vi "Fgen Module.vi"() -> ()   [LabVIEW 2021]
panel:
  in  "duration":dbl
  out "Actual Duration":dbl
  in  "I2C Generator Fgen":refnum<k15>
  in  "amplitude":dbl=6.0
  in  "frequency":dbl=6.0
  in  "waveform":T1(ring)=enum."Noise"
  in  "I2C Generator Fgen Channel":string
  out "error out":errorcluster
  in  "error in":errorcluster
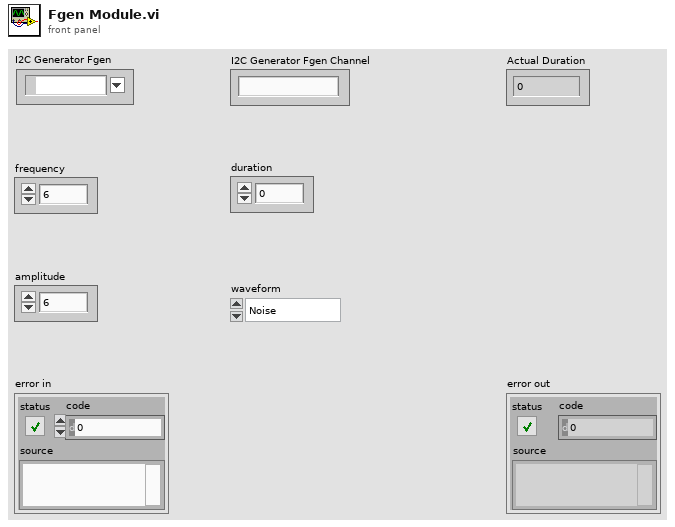
[diagram p1: front panel]
types:
  T1 = enum32{"Sine", "Square", "Triangle", "Ramp Up", "Ramp Down", "DC", "Noise", "User"}
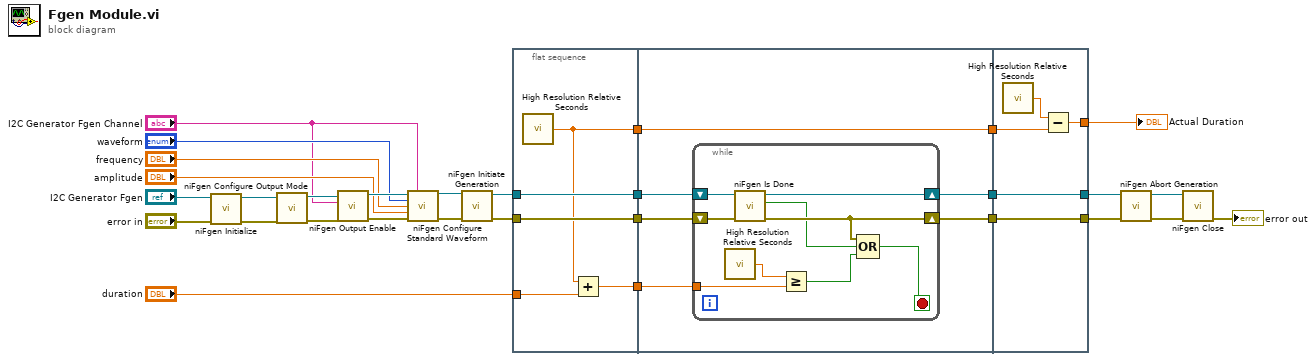
[diagram p0: block diagram]
diagram:
  n1 = call <instrlib>:"niFgen Initialize.vi"("error in (no error)"="error in", "Resource Name"="I2C Generator Fgen") -> ("error out"=w27:errorcluster, "Instrument Handle Out"=w30:refnum<k15>)  [unwired: 8 in]
  n2 = call <instrlib>:"niFgen Configure Output Mode.vi"("error in (no error)"=w27, "Instrument Handle"=w30) -> ("error out"=w15:errorcluster, "Instrument Handle Out"=w26:refnum<k15>)  [unwired: 7 in]
  n3 = call <instrlib>:"niFgen Output Enable.vi"("error in (no error)"=w15, "Channel Name"="I2C Generator Fgen Channel", "Instrument Handle"=w26) -> ("error out"=w28:errorcluster, "Instrument Handle Out"=w25:refnum<k15>)  [unwired: 7 in]
  n4 = call <instrlib>:"niFgen Configure Standard Waveform.vi"("Instrument Handle"=w25, "Channel Name"="I2C Generator Fgen Channel", "Waveform"="waveform", "Frequency"="frequency", "Amplitude"="amplitude", "error in (no error)"=w28) -> ("Instrument Handle Out"=w24:refnum<k15>, "error out"=w29:errorcluster)  [unwired: 8 in]
  n5 = call <instrlib>:"niFgen Initiate Generation.vi"("error in (no error)"=w29, "Instrument Handle"=w24) -> ("error out"=w21:errorcluster, "Instrument Handle Out"=w23:refnum<k15>)  [unwired: 8 in]
  n6 = flat-sequence {
    tunnel: w21 -> [w34]
    tunnel: w23 -> [w35]
    tunnel: [w35] -> w9
    tunnel: [w34] -> w8
    tunnel: [w33] -> w4
    tunnel: "duration" -> [w32]
    tunnel: [w31] -> w1
    tunnel: w9 -> [w41]
    tunnel: w8 -> [w39]
    tunnel: [w40] -> w7
    tunnel: [w38] -> w6
    tunnel: [w37] -> w5
    tunnel: w4 -> [w37]
    tunnel: w1 -> [w36]
    tunnel: [w54] -> w20
    tunnel: [w55] -> w22
    tunnel: w7 -> [w55]
    tunnel: w6 -> [w54]
    tunnel: w5 -> [w52]
    tunnel: [w51] -> w3
    frame #0 {
      n7 = call <vilib>:"High Resolution Relative Seconds.vi"() -> ("relative seconds"=w33:dbl)
      n8 = Add(x=w33, y=w32) -> (x+y=w31:dbl)
    }
    frame #1 {
      n9 = while {
        shift-right: [w49] -> w40
        shift-left: w41 -> [w50]
        shift-right: [w47] -> w38
        shift-left: w39 -> [w48]
        tunnel: w36 -> [w44]
        stop <- w46 stop-if-true
        n10 = call <vilib>:"High Resolution Relative Seconds.vi"() -> ("relative seconds"=w45:dbl)
        n11 = call <instrlib>:"niFgen Is Done.vi"("error in (no error)"=w48, "Instrument Handle"=w50) -> ("error out"=w47:errorcluster, "Done"=w42:bool, "Instrument Handle Out"=w49:refnum<k15>)  [unwired: 7 in]
        n12 = Greater Or Equal?(x=w45, y=w44) -> (x >= y?=w43:bool)
        n13 = Compound Arithmetic op=OR(w47, w42, w43) -> (w46:bool)
      }
    }
    frame #2 {
      n14 = call <vilib>:"High Resolution Relative Seconds.vi"() -> ("relative seconds"=w53:dbl)
      n15 = Subtract(x=w53, y=w52) -> (x-y=w51:dbl)
    }
  }
  n16 = call <instrlib>:"niFgen Abort Generation.vi"("error in (no error)"=w20, "Instrument Handle"=w22) -> ("error out"=w18:errorcluster, "Instrument Handle Out"=w19:refnum<k15>)  [unwired: 8 in]
  n17 = call <instrlib>:"niFgen Close.vi"("error in (no error)"=w18, "Instrument Handle"=w19) -> ("error out"=→"error out":errorcluster)  [unwired: 9 in]
  "Actual Duration" <- w3
